vi "Create or Add Phrase or Paragraph (Unicode).vi"(1 "Direction":enum16{"Default", "LTR", "No Bidi", "RTL"}(ring), 2 "Text":string, 3 "Paragraph indentation":T1, 7 "Paragraph refnum IN":refnum<k24>, 11 "error in (no error)":errorcluster, 12 "Font":T5={"Name"="", "Size"=-1.0, "Color"=0, "Style"={"Bold"=FALSE, "Italic"=FALSE, "Underline"=FALSE, "Strikeout"=FALSE}, "Type"={"Type&direction"=enum."Select", "Embedded"=FALSE, "Encoding"="CP1252"}}, 14 "Paragraph properties":T2) -> (4 "PDF Report duplicate":refnum<class "PDF Report Class.lvclass">, 8 "Paragraph refnum OUT":refnum<k24>, 15 "error out":errorcluster)   [LabVIEW 2019]
doc: "Version 1.0\nDeveloped by Jean-Marc Simard\nCopyright © 2010, Exaprom Inc.\nAll rights reserved.\nLicense: BSD\n\nWith iTextSharp 4.1.6 (http://itextsharp.sourceforge.net)\nunder Mozilla Public License Version 1.1\n(http://www.mozilla.org/MPL/MPL-1.1.html)"
uses:
  C:/work/niobrara_lv/labview pdf writer fixing/DLL/itextsharp.dll
  DLL/itextsharp.dll
  Controls/Text Controls/Phrase or paragraph.ctl
  LV Class/Fonts Class/Font Class.lvclass
  LV Class/PDF Report Class/PDF Report Class.lvclass
  Controls/Font Controls/Font size.ctl
  Controls/Font Controls/Font color.ctl
  Controls/Font Controls/Font complete cluster.ctl
  Controls/Text Controls/Texte alignement.ctl
  Controls/Text Controls/Line spacing.ctl
  <vilib>/Exaprom PDF/Controls/Paragraphe cluster.ctl
  Controls/Text Controls/Paragraph indentation.ctl
  Controls/Text Controls/Unicode/Type and run direction.ctl
  Controls/Font Controls/Type and encoding.ctl
panel:
  in  "PDF Report":refnum<class "PDF Report Class.lvclass">
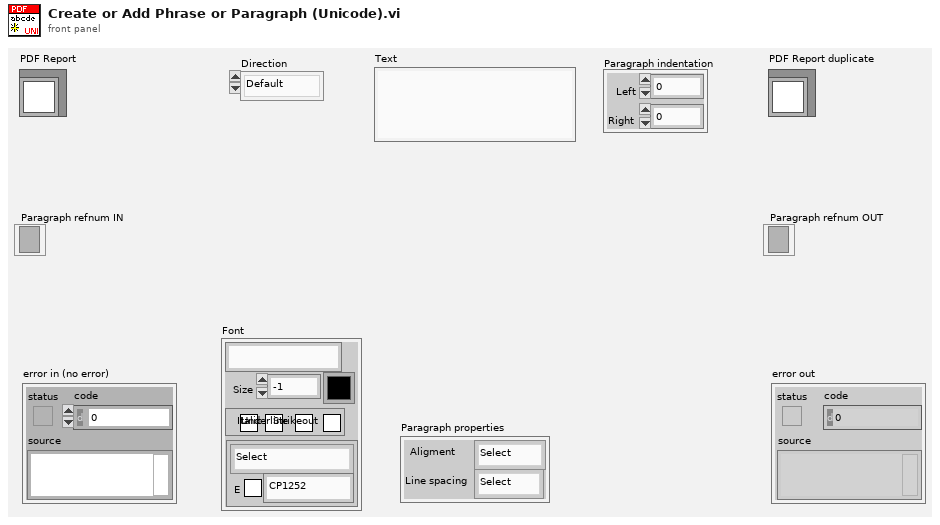
[diagram p1: front panel]
types:
  T1 = typedef "Paragraph indentation.ctl" = cluster{"Left":sgl, "Right":sgl}
  T2 = typedef "Paragraphe cluster.ctl" = cluster{" Aligment":T3, "Line spacing":T4}
  T3 = typedef "Texte alignement.ctl" = enum16{"Select", "CENTER", "JUSTIFY", "LEFT", "RIGHT"}
  T4 = typedef "Line spacing.ctl" = enum16{"Select", "1.0", "1.5", "2.0"}
  T5 = typedef "Font complete cluster.ctl" = cluster{"Name":string, "Size":T6, "Color":T7, "Style":cluster{"Bold":bool, "Italic":bool, "Underline":bool, "Strikeout":bool}, "Type":T8}
  T6 = typedef "Font size.ctl" = sgl
  T7 = typedef "Font color.ctl" = u32
  T8 = typedef "Type and encoding.ctl" = cluster{"Type&direction":T9, "Embedded":bool, "Encoding":string}
  T9 = typedef "Type and run direction.ctl" = enum16{"Select", "ASCII", "UTF-16", "UTF-16 (default)", "UTF-16 (LTR)", "UTF-16 (RTL)"}
  T10 = typedef "Phrase or paragraph.ctl" = enum16{"Add to Phrase", "Add to Paragraph", "Create Phrase", "Create Paragraph"}
  T11 = typedef "Unit.ctl" = enum16{"inch", "mm"}
  T12 = typedef "Image to Add refnum [ ].ctl" = cluster{"Image name":string, "InstanceImage":refnum<k24>}[]
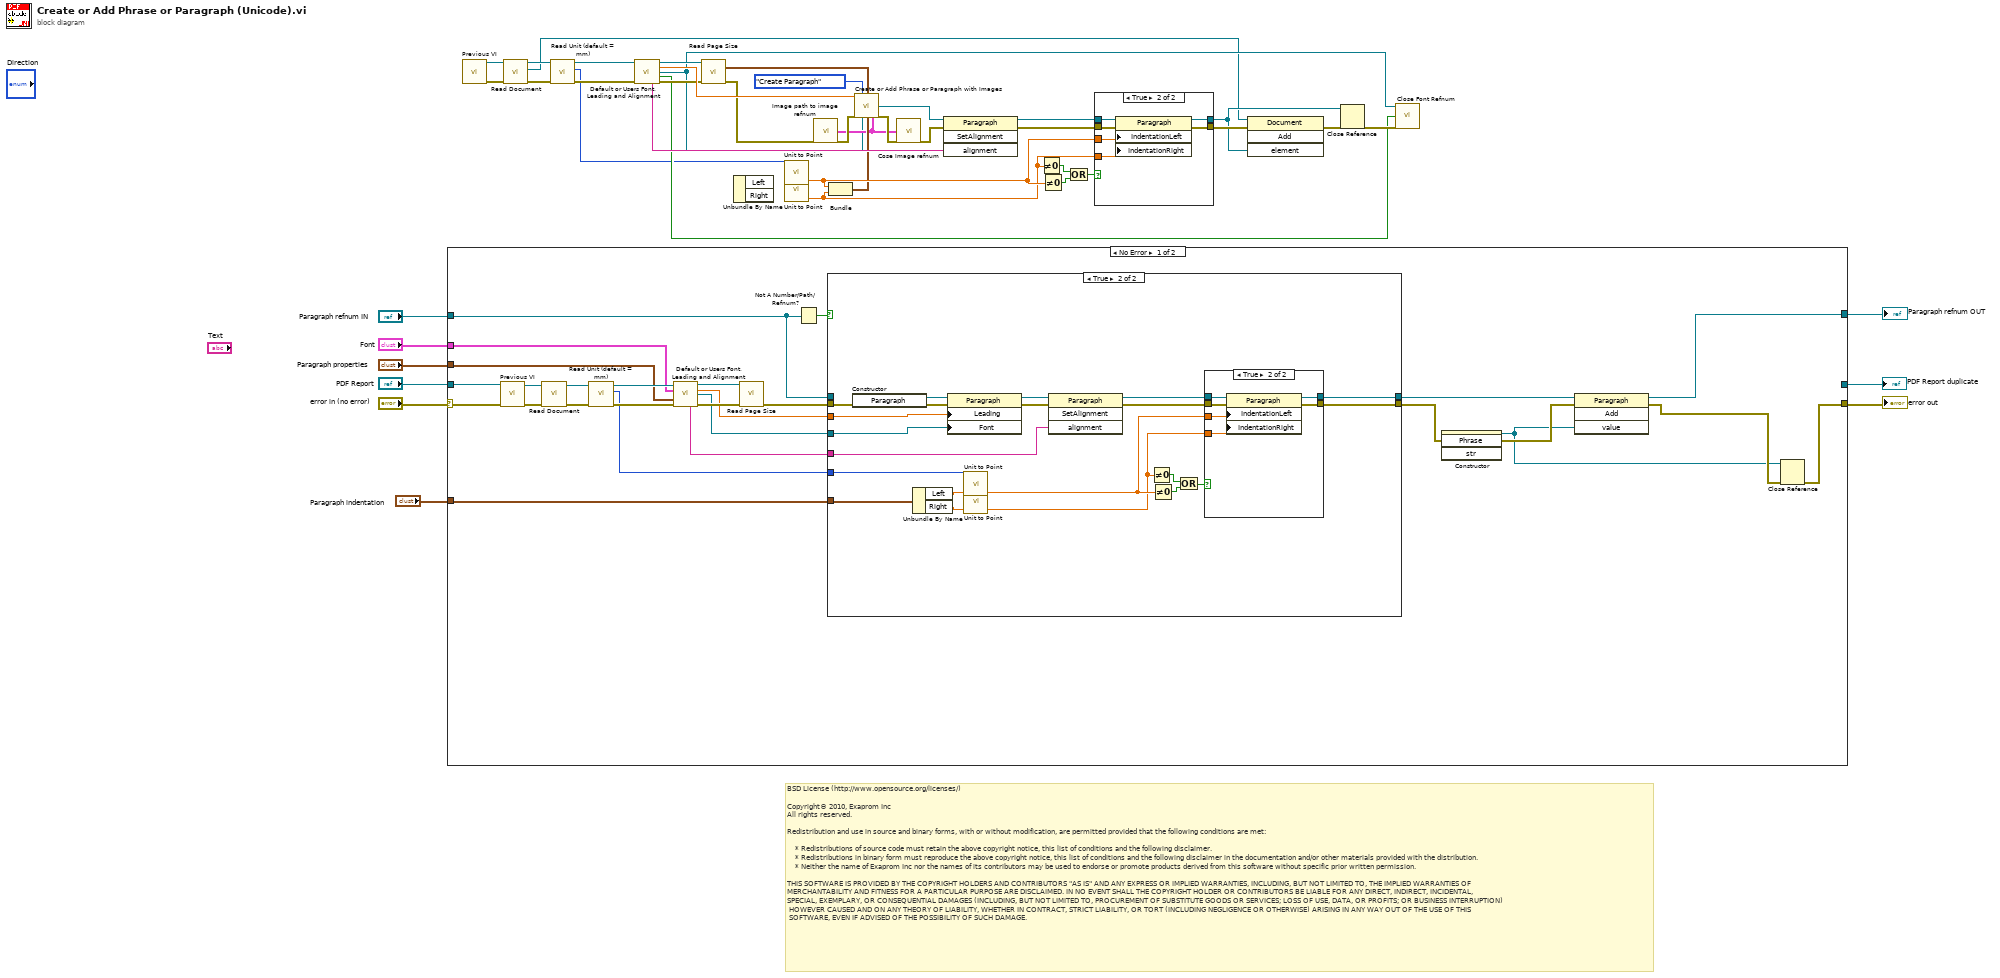
[diagram p0: block diagram]
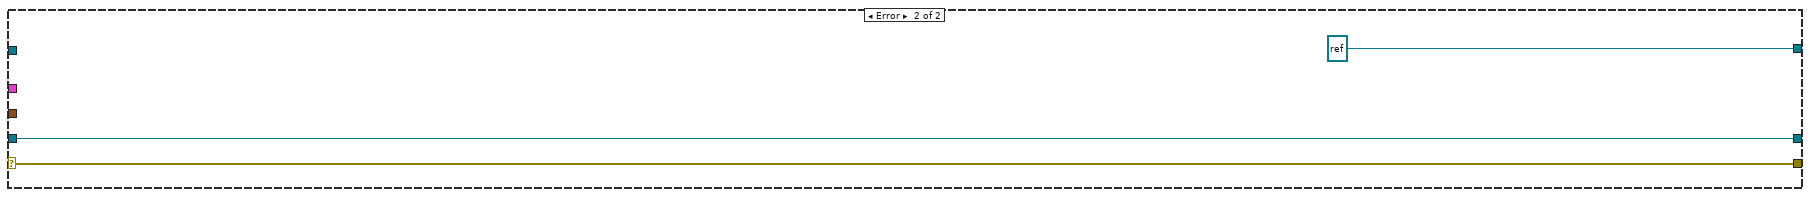
[diagram p5: hidden frame]
diagram:
  # "BSD License (http://www.opensource.org/licenses/)\n\nCopyright© 2010, Exaprom Inc\nAll rights reserved.\n\nRedistribution and use in source and binary forms, with or without modification, are permitted provided that the following conditions are met:\n\n    * Redistributions of source code must retain the above copyright notice, this list of conditions and the following disclaimer.\n    * Redistributions in binary form must reproduce the above copyright notice, this list of conditions and the following disclaimer in the documentation and/or other materials provided with the distribution.\n    * Neither the name of Exaprom Inc nor the names of its contributors may be used to endorse or promote products derived from this software without specific prior written permission.\n\nTHIS SOFTWARE IS PROVIDED BY THE COPYRIGHT HOLDERS AND CONTRIBUTORS \"AS IS\" AND ANY EXPRESS OR IMPLIED WARRANTIES, INCLUDING, BUT NOT LIMITED TO, THE IMPLIED WARRANTIES OF \nMERCHANTABILITY AND FITNESS FOR A PARTICULAR PURPOSE ARE DISCLAIMED. IN NO EVENT SHALL THE COPYRIGHT HOLDER OR CONTRIBUTORS BE LIABLE FOR ANY DIRECT, INDIRECT, INCIDENTAL,\nSPECIAL, EXEMPLARY, OR CONSEQUENTIAL DAMAGES (INCLUDING, BUT NOT LIMITED TO, PROCUREMENT OF SUBSTITUTE GOODS OR SERVICES; LOSS OF USE, DATA, OR PROFITS; OR BUSINESS INTERRUPTION)\n HOWEVER CAUSED AND ON ANY THEORY OF LIABILITY, WHETHER IN CONTRACT, STRICT LIABILITY, OR TORT (INCLUDING NEGLIGENCE OR OTHERWISE) ARISING IN ANY WAY OUT OF THE USE OF THIS\n SOFTWARE, EVEN IF ADVISED OF THE POSSIBILITY OF SUCH DAMAGE."
  n1 = case shown="No Error" "error in (no error)" {
    selector: "error in (no error)" -> [w53 w104]
    tunnel: [w69 refnum<k24> refnum ("new reference")] -> w41
    tunnel: [w68 w104] -> w42
    tunnel: "Paragraph refnum IN" -> [w62 _]
    tunnel: "PDF Report" -> [w51 w102]
    tunnel: [_ w102] -> w4
    tunnel: "Paragraph properties" -> [w50 _]
    tunnel: "Font" -> [w49 _]
    tunnel: "Paragraph indentation" -> [w45 _]
    frame No Error {
      n2 = call "Previous VI.vi"("PDF Report IN"=w51, "error in (no error)"=w53) -> ("PDF Report OUT"=w59:refnum<class "PDF Report Class.lvclass">, "error out"=w54:errorcluster)  [unwired: 12 out]
      n3 = call-dynamic "Read Document.vi"("error in (no error)"=w54, "PDF Report Class in"=w59) -> ("error out"=w57:errorcluster, "PDF Report Class out"=w60:refnum<class "PDF Report Class.lvclass">)  [unwired: 7 in, 1 out]
      n4 = call-dynamic "Read Unit (default = mm).vi"("error in (no error)"=w57, "PDF Report Class in"=w60) -> ("error out"=w58:errorcluster, "Unit (default = mm)"=w46:T11, "PDF Report Class out"=w61:refnum<class "PDF Report Class.lvclass">)  [unwired: 7 in]
      n5 = call "Default or Users Font, Leading and Alignment.vi"("PDF Report"=w61, "Font"=w49, "Paragraphe cluster"=w50, "error in (no error)"=w58) -> ("PDF Report duplicate"=w56:refnum<class "PDF Report Class.lvclass">, "Leading"=w47:T6, "Font Ref"=w48:refnum<k24>, "Aligment"=w44:string, "error out"=w55:errorcluster)  [unwired: 7 out]
      n6 = call "Read Page Size.vi"("PDF Report"=w56, "error in (no error)"=w55) -> ("error out"=w52:errorcluster)  [unwired: 13 out]
      n7 = Not A Number/Path/Refnum?(number/path/refnum=w62) -> (NaN/Path/Refnum?=w63:bool)
      n8 = case shown="True" w63 {
        tunnel: [w72 w74] -> w70
        tunnel: [w71 w73] -> w67
        tunnel: w52 -> [w71 w91]
        tunnel: w62 -> [w72 _]
        tunnel: w48 -> [_ w90]
        tunnel: w47 -> [_ w89]
        tunnel: w46 -> [_ w77]
        tunnel: w45 -> [_ w76]
        tunnel: w44 -> [_ w75]
        frame False {
        }
        frame True {
          n9 = constructor class="Paragraph"(error in=w91) -> (reference out=w92:refnum<k24>, error out=w93:errorcluster)  [unwired: 2 in, 1 out]
          n10 = Unbundle By Name(w76) -> ("Left"=w81:sgl, "Right"=w80:sgl)
          n11 = property class="Paragraph"(reference=w92, error in=w93, "Leading"=w89, "Font"=w90) -> (reference out=w83:refnum<k24>, error out=w82:errorcluster)
          n12 = call "Unit to Point.vi"("X unit"=w81, "Unit (default = mm)"=w77) -> ("X point"=w79:sgl)  [unwired: 7 out]
          n13 = call "Unit to Point.vi"("X unit"=w80, "Unit (default = mm)"=w77) -> ("X point"=w78:sgl)  [unwired: 7 out]
          n14 = invoke class="Paragraph" method="SetAlignment"(reference=w83, error in=w82, "alignment"=w75) -> (reference out=w84:refnum<k24>, error out=w85:errorcluster)  [unwired: 1 in, 2 out]
          n15 = Not Equal To 0?(x=w78) -> (x != 0?=w87:bool)
          n16 = Not Equal To 0?(x=w79) -> (x != 0?=w88:bool)
          n17 = Or(x=w87, y=w88) -> (x .or. y?=w86:bool)
          n18 = case shown="True" w86 {
            tunnel: w84 -> [w95 w101]
            tunnel: w85 -> [w94 w100]
            tunnel: [w94 w99] -> w73
            tunnel: [w95 w98] -> w74
            tunnel: w79 -> [_ w97]
            tunnel: w78 -> [_ w96]
            frame False {
            }
            frame True {
              n19 = property class="Paragraph"(reference=w101, error in=w100, "IndentationLeft"=w97, "IndentationRight"=w96) -> (reference out=w98:refnum<k24>, error out=w99:errorcluster)
            }
          }
        }
      }
      n20 = constructor class="Phrase"(error in=w67) -> (reference out=w64:refnum<k24>, error out=w66:errorcluster)  [unwired: 3 in, 2 out]
      n21 = invoke class="Paragraph" method="Add"(reference=w70, error in=w66, "value"=w64) -> (reference out=w69:refnum<k24>, error out=w65:errorcluster)  [unwired: 1 in, 2 out]
      n22 = Close Reference(reference=w64, error in (no error)=w65) -> (error out=w68:errorcluster)
    }
    frame Error {
    }
  }
  "error out" <- w42
  "Paragraph refnum OUT" <- w41
  "PDF Report duplicate" <- w4
  n23 = call "Previous VI.vi"() -> ("PDF Report OUT"=w10:refnum<class "PDF Report Class.lvclass">, "error out"=w22:errorcluster)  [unwired: 2 in, 12 out]
  n24 = call-dynamic "Read Document.vi"("error in (no error)"=w22, "PDF Report Class in"=w10) -> ("error out"=w12:errorcluster, "Document"=w6:refnum<k24>, "PDF Report Class out"=w9:refnum<class "PDF Report Class.lvclass">)  [unwired: 7 in]
  n25 = call-dynamic "Read Unit (default = mm).vi"("error in (no error)"=w12, "PDF Report Class in"=w9) -> ("error out"=w11:errorcluster, "Unit (default = mm)"=w7:T11, "PDF Report Class out"=w8:refnum<class "PDF Report Class.lvclass">)  [unwired: 7 in]
  n26 = call "Default or Users Font, Leading and Alignment.vi"("PDF Report"=w8, "error in (no error)"=w11) -> ("PDF Report duplicate"=w18:refnum<class "PDF Report Class.lvclass">, "Leading"=w29:T6, "Font Ref"=w13:refnum<k24>, "Close Font Ref"=w14:bool, "Aligment"=w37:string, "error out"=w20:errorcluster)  [unwired: 2 in, 6 out]
  n27 = call "Read Page Size.vi"("PDF Report"=w18, "error in (no error)"=w20) -> ("Text zone (points)"=w21:cluster{"widht":sgl, "height":sgl}, "error out"=w19:errorcluster)  [unwired: 12 out]
  n28 = Unbundle By Name() -> ()  [unwired: 1 in, 2 out]
  n29 = call "Unit to Point.vi"("Unit (default = mm)"=w7) -> ("X point"=w27:sgl)  [unwired: 1 in, 7 out]
  n30 = call "Unit to Point.vi"("Unit (default = mm)"=w7) -> ("X point"=w26:sgl)  [unwired: 1 in, 7 out]
  n31 = call "Image path to image refnum.vi"("error in (no error)"=w19) -> ("Image to Add refnum [ ]"=w17:T12, "error out"=w39:errorcluster)  [unwired: 3 in, 10 out]
  n32 = Bundle("X point"=w27, "X point"=w26) -> (w25:cluster{" X point":sgl, " X point":sgl})  [unwired: 1 out]
  n33 = call "Create or Add Phrase or Paragraph with Images.vi"("Leading"=w29, "Phrase or paragraph"=Phrase_or_paragraph."Create Paragraph", "Text zone (points)"=w21, "error in (no error)"=w39, "Font refnum"=w13, "Paragraph indentation (points)"=w25, "Image to Add refnum [ ]"=w17) -> ("Paragraph refnum OUT"=w28:refnum<k24>, "error out"=w24:errorcluster)  [unwired: 4 in, 3 out]
  n34 = call "Cose Image refnum.vi"("Image to Add refnum [ ]"=w17, "error in (no error)"=w24) -> ("error out"=w23:errorcluster)  [unwired: 13 out]
  n35 = invoke class="Paragraph" method="SetAlignment"(reference=w28, error in=w23, "alignment"=w37) -> (reference out=w36:refnum<k24>, error out=w35:errorcluster)  [unwired: 1 in, 2 out]
  n36 = Not Equal To 0?(x=w26) -> (x != 0?=w31:bool)
  n37 = Not Equal To 0?(x=w27) -> (x != 0?=w30:bool)
  n38 = Or(x=w31, y=w30) -> (x .or. y?=w32:bool)
  n39 = case shown="True" w32 {
    tunnel: w36 -> [w106 w112]
    tunnel: w35 -> [w105 w111]
    tunnel: [w105 w110] -> w34
    tunnel: [w106 w109] -> w33
    tunnel: w27 -> [_ w108]
    tunnel: w26 -> [_ w107]
    frame False {
    }
    frame True {
      n40 = property class="Paragraph"(reference=w112, error in=w111, "IndentationLeft"=w108, "IndentationRight"=w107) -> (reference out=w109:refnum<k24>, error out=w110:errorcluster)
    }
  }
  n41 = invoke class="Document" method="Add"(reference=w6, error in=w34, "element"=w33) -> (error out=w16:errorcluster)  [unwired: 1 in, 3 out]
  n42 = Close Reference(reference=w33, error in (no error)=w16) -> (error out=w15:errorcluster)
  n43 = call "Close Font Refnum.vi"("Font Refnum"=w13, "Close ?"=w14, "error in (no error)"=w15) -> ()  [unwired: 12 in, 1 out]
